vi "Q3 top level.vi"() -> ()   [LabVIEW 2014]
panel:
  out "Array":dbl[][](array[numeric])
  in  "lower bound":dbl
  in  "upper bound":dbl
  # "index"
  # "id"
  # "score"
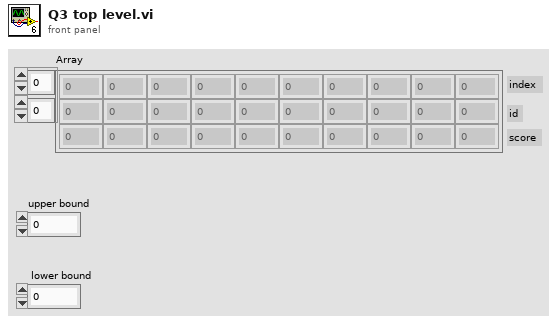
[diagram p1: front panel]
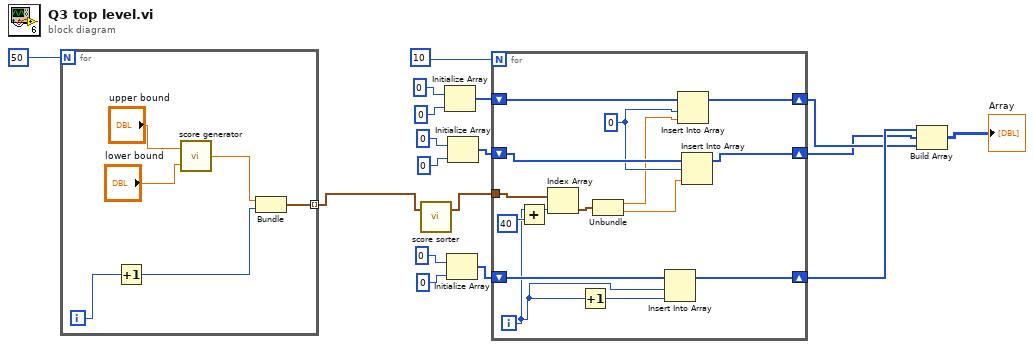
[diagram p0: block diagram]
diagram:
  n1 = for {
    N: 50 -> [_]
    tunnel: [w18] -> w15 mode=indexing
    i -> [w21]
    n2 = Increment(x=w21) -> (x+1=w19:i32)
    n3 = call "score generator.vi"("Numeric 2"="lower bound", "Numeric"="upper bound") -> ("Numeric 3"=w20:dbl)
    n4 = Bundle("Numeric 3"=w20, w19) -> (w18:cluster{"Numeric 3":dbl, i32})  [unwired: 1 in]
  }
  n5 = call "score sorter.vi"("Array 2"=w15) -> ("Array"=w14:cluster{"Numeric":dbl, "Numeric 2":dbl}[])  [unwired: 2 in]
  n6 = Initialize Array(0, 0) -> (w7:i32[])
  n7 = Initialize Array(0, 0) -> (w5:i32[])
  n8 = Initialize Array(0, 0) -> (w6:i32[])
  n9 = for {
    N: 10 -> [_]
    tunnel: w14 -> [w38]
    shift-right: [w31] -> w2
    shift-left: w7 -> [w34]
    shift-right: [w32] -> w1
    shift-left: w6 -> [w33]
    shift-right: [w26] -> w4
    shift-left: w5 -> [w27]
    i -> [w24]
    w30 = 0
    n10 = Add(x=w24, y=40) -> (x+y=w36:i32)
    n11 = Index Array(array=w38, index=w36) -> (element=w37:cluster{"Numeric":dbl, "Numeric 2":dbl})
    n12 = Increment(x=w24) -> (x+1=w25:i32)
    n13 = Unbundle(w37) -> ("Numeric"=w29:dbl, "Numeric 2"=w28:dbl)
    n14 = Insert Into Array(array=w27, index=w24, new element=w25) -> (w26:i32[])
    n15 = Insert Into Array(array=w34, index=w30, new element=w29) -> (w31:i32[])
    n16 = Insert Into Array(array=w33, index=w30, new element=w28) -> (w32:i32[])
  }
  n17 = Build Array(w4, w1, w2) -> (→"Array":i32[][])
